vi "WriteErrorReport.vi"(7 "StepName":string, 9 "message":string, 10 "source out":string, 11 "Error":bool) -> ()   [LabVIEW 2013]
uses:
  <vilib>/Utility/error.llb/DialogType.ctl
  GlobValue.vi
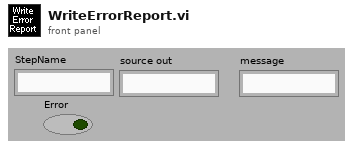
[diagram p1: front panel]
types:
  T1 = enum16{"open", "replace", "create", "open or create", "replace or create", "replace or create with confirmation"}
  T2 = typedef "DialogType.ctl" = u16
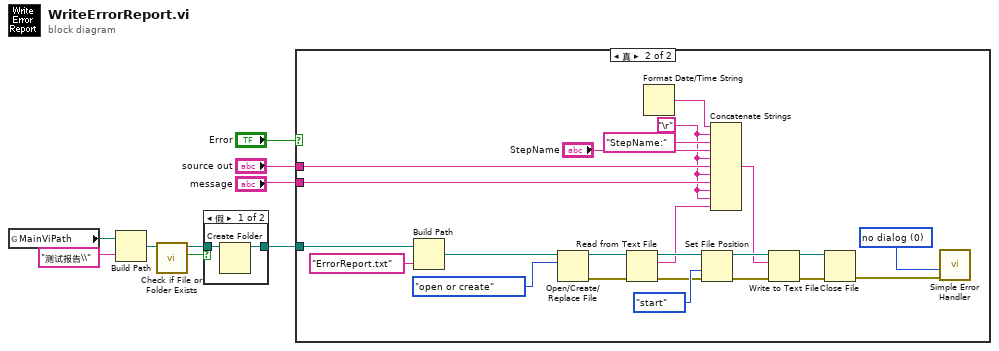
[diagram p0: block diagram]
diagram:
  n1 = global read "GlobValue.vi" "MainViPath"() -> (w1:path)
  n2 = Build Path(base path=w1, name or relative path="测试报告\\" ("名称或相对路径")) -> (appended path=w2:path)
  n3 = call <vilib>:"Check if File or Folder Exists.vi"("path"=w2) -> ("file or folder exists?"=w6:bool, "dup path"=w5:path)  [unwired: 8 in, 1 out]
  n4 = case shown="假" w6 {
    tunnel: w5 -> [w11 w12]
    tunnel: [w10 w12] -> w4
    frame False {
      n5 = Create Folder(path (use dialog)=w11) -> (created path=w10:path)  [unwired: 2 in, 2 out]
    }
    frame True {
    }
  }
  n6 = case shown="真" "Error" {
    tunnel: "source out" -> [_ w28]
    tunnel: "message" -> [_ w26]
    tunnel: w4 -> [_ w13]
    frame False {
    }
    frame True {
      w14 = T2 0 items=["no dialog", "OK message", "continue or stop message", "OK message + warnings", "continue/stop + warnings"] ("type of dialog (OK msg:1)")
      w18 = "\r"
      n7 = Build Path(base path=w13, name or relative path="ErrorReport.txt" ("名称或相对路径")) -> (appended path=w16:path)
      n8 = Open/Create/Replace File(file path (use dialog)=w16, operation (0:open)=T1."open or create" ("操作(0:open)")) -> (refnum out=w23:refnum<file>, error out=w22:errorcluster)  [unwired: 1 in, 4 out]
      n9 = Read from Text File(file (use dialog)=w23, error in=w22) -> (refnum out=w21:refnum<file>, text=w19:string, error out=w20:errorcluster)  [unwired: 3 out]
      n10 = Format Date/Time String() -> (date/time string=w29:string)  [unwired: 3 out]
      n11 = Set File Position(refnum=w21, from (0:start)=enum16{"start", "end", "current"}."start" ("自（0:起始）"), error in=w20) -> (refnum out=w35:refnum<file>, error out=w33:errorcluster)  [unwired: 1 out]
      n12 = Concatenate Strings(w29, w18, "StepName:" ("字符串"), "StepName", w18, w28, w18, w26, w18, w18, w19) -> (w27:string)
      n13 = Write to Text File(file (use dialog)=w35, text=w27, error in=w33) -> (refnum out=w30:refnum<file>, error out=w31:errorcluster)  [unwired: 2 out]
      n14 = Close File(refnum=w30, error in=w31) -> (error out=w15:errorcluster)  [unwired: 1 out]
      n15 = call <vilib>:"Simple Error Handler.vi"("type of dialog (OK msg:1)"=w14, "error in (no error)"=w15) -> ()  [unwired: 3 in, 5 out]
    }
  }
